vi "SmartSEM Remote API FIB mag.vi"(8 "error in":errorcluster, 10 "FIB FOV (um)":sgl=500.0 format="%.3g", 11 "ActiveX Container":refnum<k7>(container)) -> (0 "error out":errorcluster, 3 "reference out":refnum<k7>)   [LabVIEW 2018]
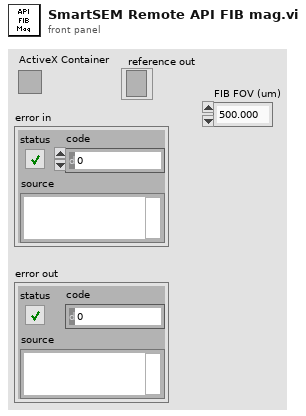
[diagram p1: front panel]
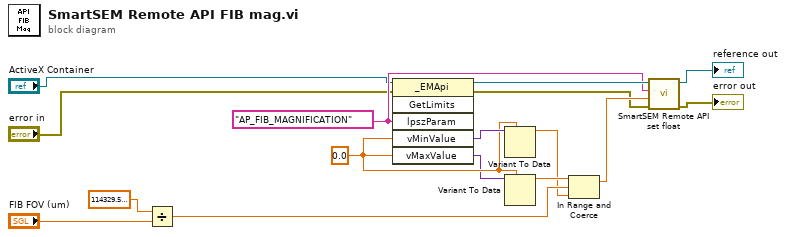
[diagram p0: block diagram]
diagram:
  w15 = sgl 0.0
  w7 = "AP_FIB_MAGNIFICATION" ("lpszParam")
  n1 = Divide(x=sgl 114329.59, y="FIB FOV (um)") -> (x/y=w12:sgl)
  n2 = invoke class="_EMApi" method="GetLimits"(reference="ActiveX Container", error in="error in", "lpszParam"=w7, "vMinValue"=w15, "vMaxValue"=w15) -> (reference out=w8:refnum<k7>, error out=w5:errorcluster, "vMinValue"=w16:variant, "vMaxValue"=w9:variant)  [unwired: 1 in, 2 out]
  n3 = Variant To Data(type=w15, Variant=w16) -> (data=w10:sgl)  [unwired: 1 in, 1 out]
  n4 = Variant To Data(type=w15, Variant=w9) -> (data=w11:sgl)  [unwired: 1 in, 1 out]
  n5 = In Range and Coerce(upper limit=w11, x=w12, lower limit=w10) -> (coerced(x)=w6:sgl)  [unwired: 1 out]
  n6 = call "SmartSEM Remote API set float.vi"("error in"=w5, "vValue"=w6, "lpszParam"=w7, "ActiveX Container"=w8) -> ("error out"=→"error out":errorcluster, "reference out"=→"reference out":refnum<k7>)  [unwired: 6 in]
